vi "MecaKinematics_ToWheelSpeeds.vi"(9 "CenterOfRotation":T2 {"Y" format="%14.3f"; "X" format="%14.3f"}, 10 "ChassisSpeeds":T5 {"vOmega" format="%10.3f"; "vY" format="%10.3f"; "vX" format="%10.3f"}, 11 "in MECA_DRIVE_KINEMATICS":T1={"FrontLeft"={"X"=0.0, "Y"=0.0}, "FrontRight"={"X"=0.0, "Y"=0.0}, "RearLeft"={"X"=0.0, "Y"=0.0}, "RearRight"={"X"=0.0, "Y"=0.0}, "InverseKinematics"=[[0.0, 1.0, -1.0, 0.0], [0.0, 1.0, 1.0, 0.0], [0.0, 1.0, 1.0, 0.0], [0.0, 1.0, -1.0, 0.0]], "ForwardKinematics"=[[0.0, 1.0, -1.0, 0.0], [0.0, 1.0, 1.0, 0.0], [0.0, 1.0, 1.0, 0.0], [0.0, 1.0, -1.0, 0.0]], "PrevCoR"={"X"=0.0, "Y"=0.0}} {"PrevCoR"."Y" format="%14.3f"; "PrevCoR"."X" format="%14.3f"; "RearRight"."Y" format="%14.3f"; "RearRight"."X" format="%14.3f"; "RearLeft"."Y" format="%14.3f"; "RearLeft"."X" format="%14.3f"; "FrontRight"."Y" format="%14.3f"; "FrontRight"."X" format="%14.3f"; "FrontLeft"."Y" format="%14.3f"; "FrontLeft"."X" format="%14.3f"}) -> (1 "MECA_WHEEL_SPEEDS":T4 {"RearRightSpeed" format="%19.3f"; "RearLeftSpeed" format="%19.3f"; "FrontRightSpeed" format="%19.3f"; "FrontLeftSpeed" format="%19.3f"}, 3 "out MECA_DRIVE_KINEMATICS":T1={"FrontLeft"={"X"=0.0, "Y"=0.0}, "FrontRight"={"X"=0.0, "Y"=0.0}, "RearLeft"={"X"=0.0, "Y"=0.0}, "RearRight"={"X"=0.0, "Y"=0.0}, "InverseKinematics"=[[0.0, 1.0, -1.0, 0.0], [0.0, 1.0, 1.0, 0.0], [0.0, 1.0, 1.0, 0.0], [0.0, 1.0, -1.0, 0.0]], "ForwardKinematics"=[[0.0, 1.0, -1.0, 0.0], [0.0, 1.0, 1.0, 0.0], [0.0, 1.0, 1.0, 0.0], [0.0, 1.0, -1.0, 0.0]], "PrevCoR"={"X"=0.0, "Y"=0.0}} {"PrevCoR"."Y" format="%14.3f"; "PrevCoR"."X" format="%14.3f"; "RearRight"."Y" format="%14.3f"; "RearRight"."X" format="%14.3f"; "RearLeft"."Y" format="%14.3f"; "RearLeft"."X" format="%14.3f"; "FrontRight"."Y" format="%14.3f"; "FrontRight"."X" format="%14.3f"; "FrontLeft"."Y" format="%14.3f"; "FrontLeft"."X" format="%14.3f"})   [LabVIEW 2019, in "Trajectory_Library.lvlib"]
doc: "Performs inverse kinematics to return the wheel speeds from a desired chassis velocity. This method is often used to convert joystick values into wheel speeds.\n \nThis function also supports variable centers of rotation. During normal operations, the center of rotation is usually the same as the physical center of the robot; therefore, the argument is defaulted to that use case. However, if you wish to change the center of rotation for evasive manuevers, vision alignment, or for any other use case, you can do so.\n \nParameters:\n - MecaDriveKinematics - Data structure\n - chassisSpeeds - The desired chassis speed.\n - centerOfRotation - The center of rotation. For example, if you set the center of rotation at one corner of the robot and provide a chassis speed that only has a dtheta component, the robot will rotate around that corner. (Meters)\n\nReturns:\n - MecaDriveKinematics - Updated data structure\n - WheelSpeeds - The wheel speeds. Use caution because they are not normalized. Sometimes, a user input may cause one of the wheel speeds to go above the attainable max velocity. Use the MecaWheel_normalize function to rectify this issue."
uses:
  Trajectory_Library.lvlib
  TRANSLATION2D.ctl
  CHASSIS_SPEEDS.ctl
  MECA_WHEEL_SPEEDS.ctl
  MECA_DRIVE_KINEMATICS.ctl
  <vilib>/Analysis/Matrix/Datatypes/RealMatrix.ctl
  Translation_Create.vi
  <vilib>/Analysis/Matrix/Numeric/Multiply/Multiply - RM,RM.vi
  <vilib>/Analysis/Matrix/NI_Matrix.lvlib
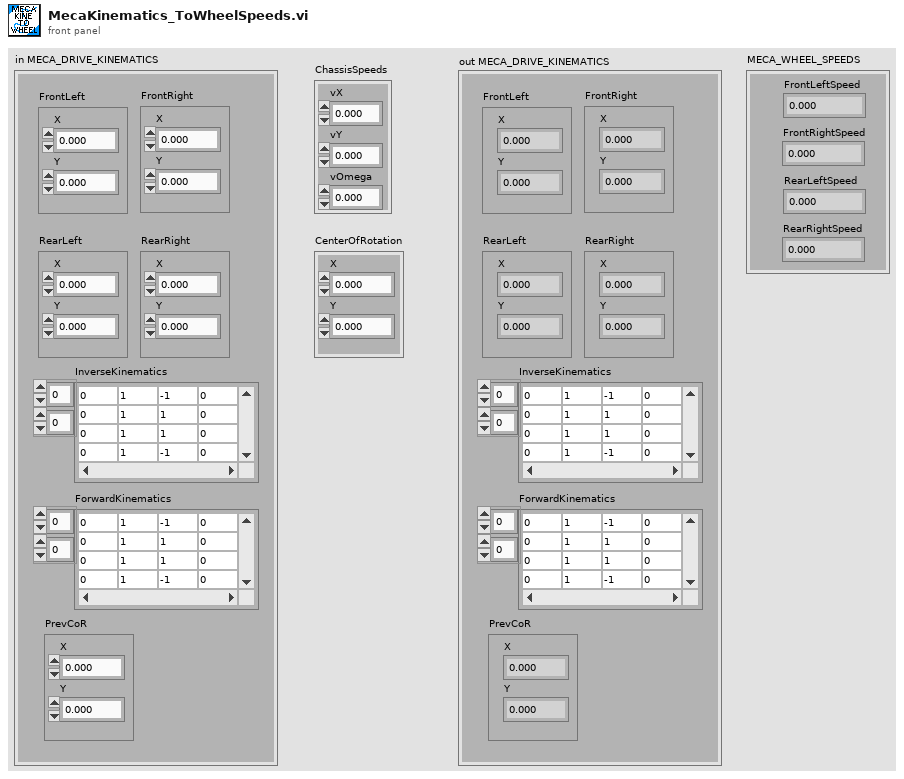
[diagram p1: front panel]
types:
  T1 = typedef "Trajectory_Library.lvlib/MECA_DRIVE_KINEMATICS.ctl" = cluster{"FrontLeft":T2, "FrontRight":T2, "RearLeft":T2, "RearRight":T2, "InverseKinematics":T3, "ForwardKinematics":T3, "PrevCoR":T2}
  T2 = typedef "Trajectory_Library.lvlib/TRANSLATION2D.ctl" = cluster{"X":dbl, "Y":dbl}
  T3 = typedef "NI_Matrix.lvlib/RealMatrix.ctl" = dbl[][]
  T4 = typedef "Trajectory_Library.lvlib/MECA_WHEEL_SPEEDS.ctl" = cluster{"FrontLeftSpeed":dbl, "FrontRightSpeed":dbl, "RearLeftSpeed":dbl, "RearRightSpeed":dbl}
  T5 = typedef "Trajectory_Library.lvlib/CHASSIS_SPEEDS.ctl" = cluster{"vX":dbl, "vY":dbl, "vOmega":dbl}
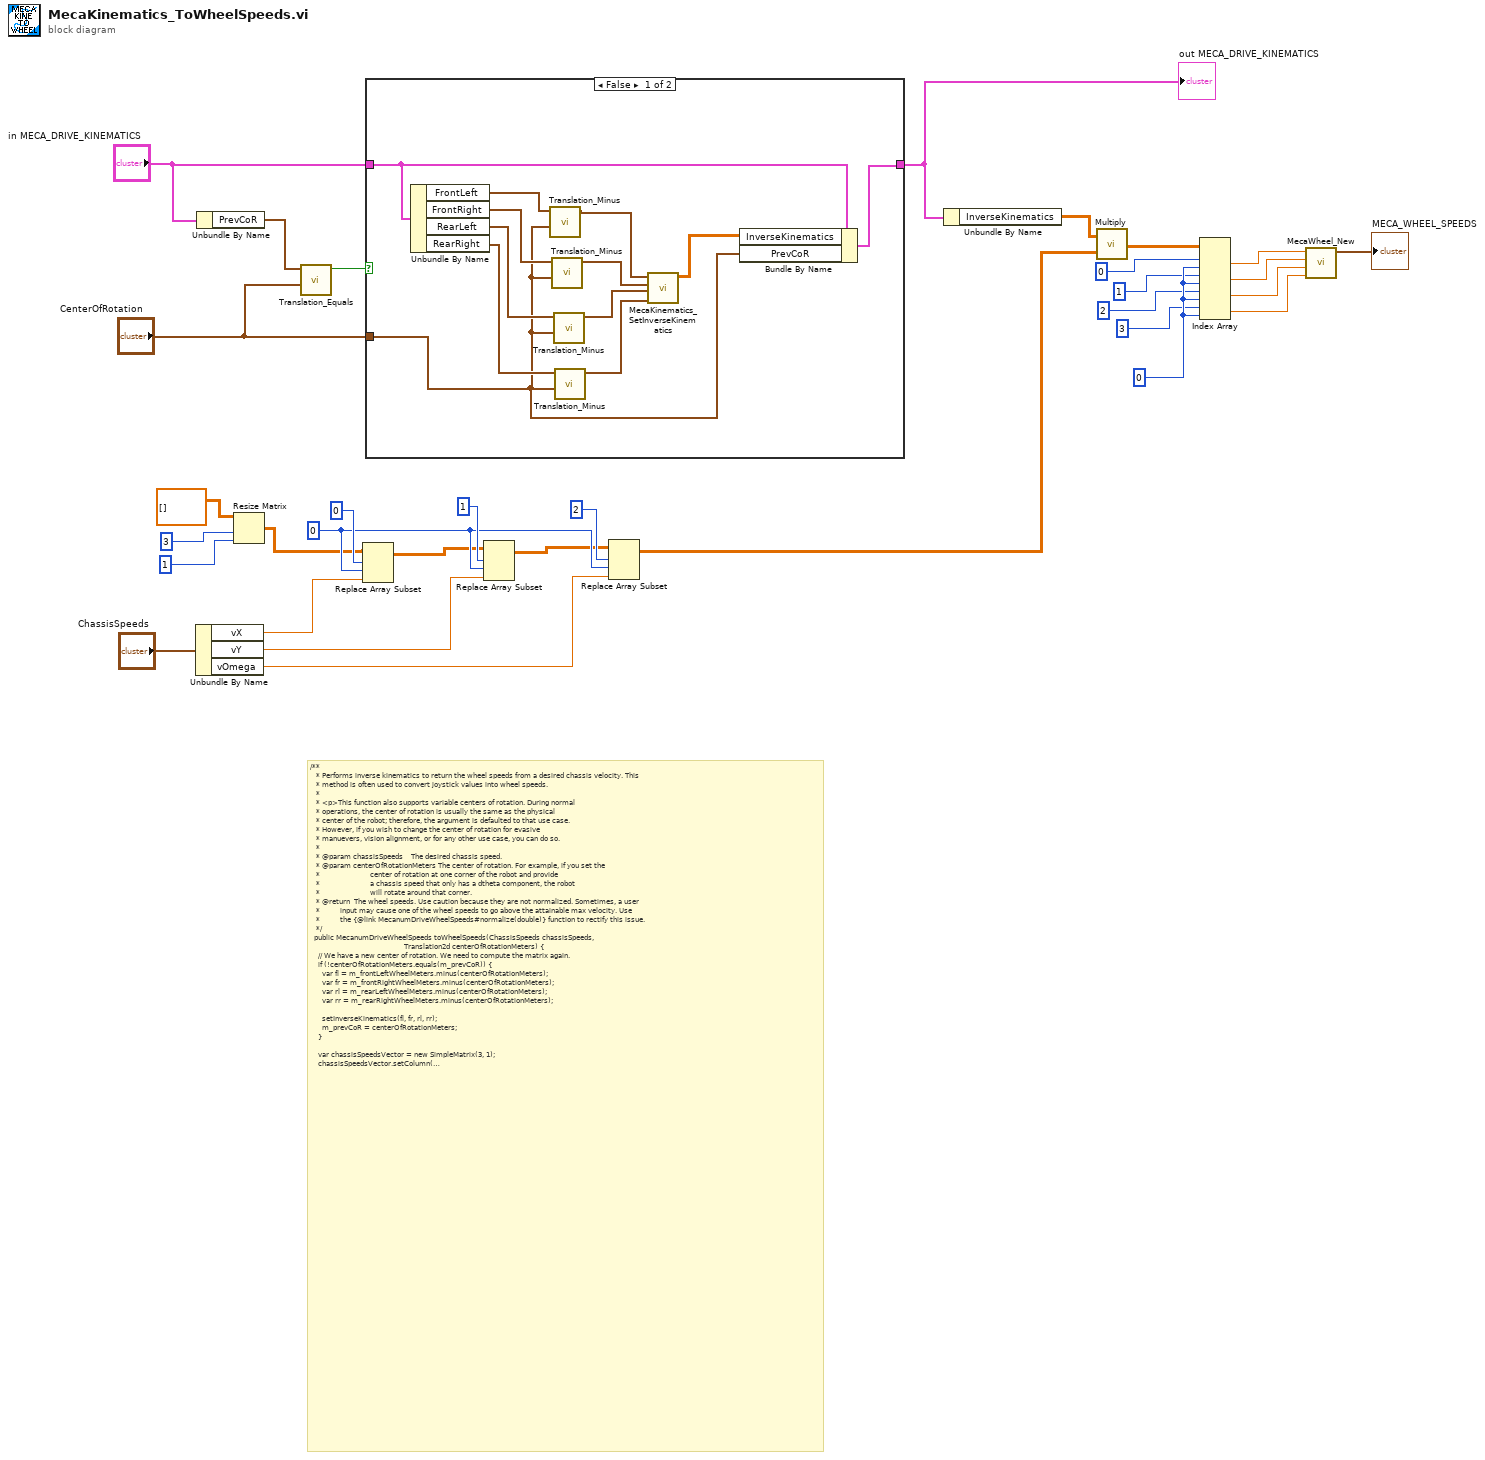
[diagram p0: block diagram]
diagram:
  w10 = 0 ("index (col)")
  w23 = 0 ("disabled index (col)")
  # "/**\n   * Performs inverse kinematics to return the wheel speeds from a desired chassis velocity. This\n   * method is often used to convert joystick values into wheel speeds.\n   *\n   * <p>This function also supports variable centers of rotation. During normal\n   * operations, the center of rotation is usually the same as the physical\n   * center of the robot; therefore, the argument is defaulted to that use case.\n   * However, if you wish to change the center of rotation for evasive\n   * manuevers, vision alignment, or for any other use case, you can do so.\n   *\n   * @param chassisSpeeds    The desired chassis speed.\n   * @param centerOfRotationMeters The center of rotation. For example, if you set the\n   *                         center of rotation at one corner of the robot and provide\n   *                         a chassis speed that only has a dtheta component, the robot\n   *                         will rotate around that corner.\n   * @return  The wheel speeds. Use caution because they are not normalized. Sometimes, a user\n   *          input may cause one of the wheel speeds to go above the attainable max velocity. Use\n   *          the {@link MecanumDriveWheelSpeeds#normalize(double)} function to rectify this issue.\n   */\n  public MecanumDriveWheelSpeeds toWheelSpeeds(ChassisSpeeds chassisSpeeds,\n                                               Translation2d centerOfRotationMeters) {\n    // We have a new center of rotation. We need to compute the matrix again.\n    if (!centerOfRotationMeters.equals(m_prevCoR)) {\n      var fl = m_frontLeftWheelMeters.minus(centerOfRotationMeters);\n      var fr = m_frontRightWheelMeters.minus(centerOfRotationMeters);\n      var rl = m_rearLeftWheelMeters.minus(centerOfRotationMeters);\n      var rr = m_rearRightWheelMeters.minus(centerOfRotationMeters);\n\n      setInverseKinematics(fl, fr, rl, rr);\n      m_prevCoR = centerOfRotationMeters;\n    }\n\n    var chassisSpeedsVector = new SimpleMatrix(3, 1);\n    chassisSpeedsVector.setColumn(0, 0,\n        chassisSpeeds.vxMetersPerSecond, chassisSpeeds.vyMetersPerSecond,\n        chassisSpeeds.omegaRadiansPerSecond);\n\n    var wheelsMatrix = m_inverseKinematics.mult(chassisSpeedsVector);\n    return new MecanumDriveWheelSpeeds(\n        wheelsMatrix.get(0, 0),\n        wheelsMatrix.get(1, 0),\n        wheelsMatrix.get(2, 0),\n        wheelsMatrix.get(3, 0)\n    );\n  }"
  n1 = Unbundle By Name("ChassisSpeeds") -> ("vX"=w21:dbl, "vY"=w20:dbl, "vOmega"=w19:dbl)
  n2 = Unbundle By Name("in MECA_DRIVE_KINEMATICS") -> ("PrevCoR"=w32:T2)
  n3 = Resize Matrix(1:1 ("number of columns"), 2:3 ("number of rows"), 4:T3 [] ("matrix")) -> (0:w18:T3)
  n4 = call "Translation_Equals.vi"("other Translation"="CenterOfRotation", "In Translation"=w32) -> ("Equals"=w31:bool)  [unwired: 9 in]
  n5 = Replace Array Subset(array=w18, new element=w21, index (row)=0 ("disabled index (row)"), index (col)=w23) -> (w17:T3)
  n6 = case shown="False" w31 {
    tunnel: "in MECA_DRIVE_KINEMATICS" -> [w36 w45]
    tunnel: [w35 w45] -> w15
    tunnel: "CenterOfRotation" -> [w33 _]
    frame False {
      n7 = Unbundle By Name(w36) -> ("FrontLeft"=w44:T2, "FrontRight"=w43:T2, "RearLeft"=w42:T2, "RearRight"=w41:T2)
      n8 = call "Translation_Minus.vi"("other Translation"=w33, "In Translation"=w44) -> ("Out Translation"=w40:T2)  [unwired: 9 in]
      n9 = call "Translation_Minus.vi"("other Translation"=w33, "In Translation"=w43) -> ("Out Translation"=w39:T2)  [unwired: 9 in]
      n10 = call "Translation_Minus.vi"("other Translation"=w33, "In Translation"=w42) -> ("Out Translation"=w38:T2)  [unwired: 9 in]
      n11 = call "Translation_Minus.vi"("other Translation"=w33, "In Translation"=w41) -> ("Out Translation"=w37:T2)  [unwired: 9 in]
      n12 = call "MecaKinematics_SetInverseKinematics.vi"("RearRight"=w37, "RearLeft"=w38, "FrontRight"=w39, "FrontLeft"=w40) -> ("InverseKinematics"=w34:T3)  [unwired: 7 in]
      n13 = Bundle By Name(cluster=w36, "InverseKinematics"=w34, "PrevCoR"=w33) -> (w35:T1)
    }
    frame True {
    }
  }
  "out MECA_DRIVE_KINEMATICS" <- w15
  n14 = Replace Array Subset(array=w17, new element=w20, index (row)=1 ("disabled index (row)"), index (col)=w23) -> (w16:T3)
  n15 = Replace Array Subset(array=w16, new element=w19, index (row)=2 ("disabled index (row)"), index (col)=w23) -> (w13:T3)
  n16 = Unbundle By Name(w15) -> ("InverseKinematics"=w14:T3)
  n17 = call-poly <vilib>:"Multiply.vi"("Real Matrix B"=w13, "Real Matrix A"=w14) -> ("A * B"=w11:T3)
  n18 = Index Array(array=w11, index (row) #1=0 ("index (row)"), index (col) #1=w10, index (row) #2=1 ("index (row)"), index (col) #2=w10, index (row) #3=2 ("index (row)"), index (col) #3=w10, index (row) #4=3 ("index (row)"), index (col) #4=w10) -> (element #1=w5:dbl, element #2=w4:dbl, element #3=w3:dbl, element #4=w2:dbl)
  n19 = call "MecaWheel_New.vi"("RearRightSpeed"=w2, "RearLeftSpeed"=w3, "FrontRightSpeed"=w4, "FrontLeftSpeed"=w5) -> ("MECA_WHEEL_SPEEDS"=→"MECA_WHEEL_SPEEDS":T4)  [unwired: 7 in]
